vi "Read OPC UA to Azure SQL.vi"() -> ()   [LabVIEW 2019]
uses:
  <vilib>/OPCUA/client/Multiple Read Double.vi
  <vilib>/OPCUA/NI OPC UA Client.lvlib
panel:
  in  "SQL Connection string":string="PROVIDER=SQLOLEDB;DATA SOURCE=tcp:220888.database.windows.net;UID=haavardnk;PWD=Password123;DATABASE=Lab1"
  out "Temperature Value":dbl=24.475354555818342
  in  "Server Endpoint URL":string="opc.tcp://DESKTOP-2K1CGSL:49580"
  in  "stop":bool
  in  "Node Id":string="ns=2;s=Process Data.Temperature"
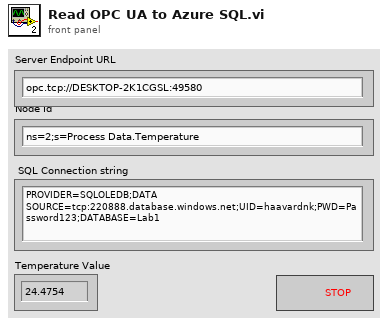
[diagram p1: front panel]
types:
  T1 = cluster{"message mode":enum16{"None", "Sign", "Sign and Encrypt"}, "security":enum16{"Basic256", "Basic128Rsa15"}}
  T2 = typedef "OPC UA Client Refnum.ctl" = refnum<k21>
  T3 = typedef "NodeId.ctl" = string
  T4 = typedef "OPC UA StatusCode.ctl" = u32
  T5 = cluster{"node ID":T3, "value ":dbl, "timestamp":timestamp, "status":T4}[]
  T6 = cluster{"node ID":T3, "value ":dbl, "timestamp":timestamp, "status":T4}
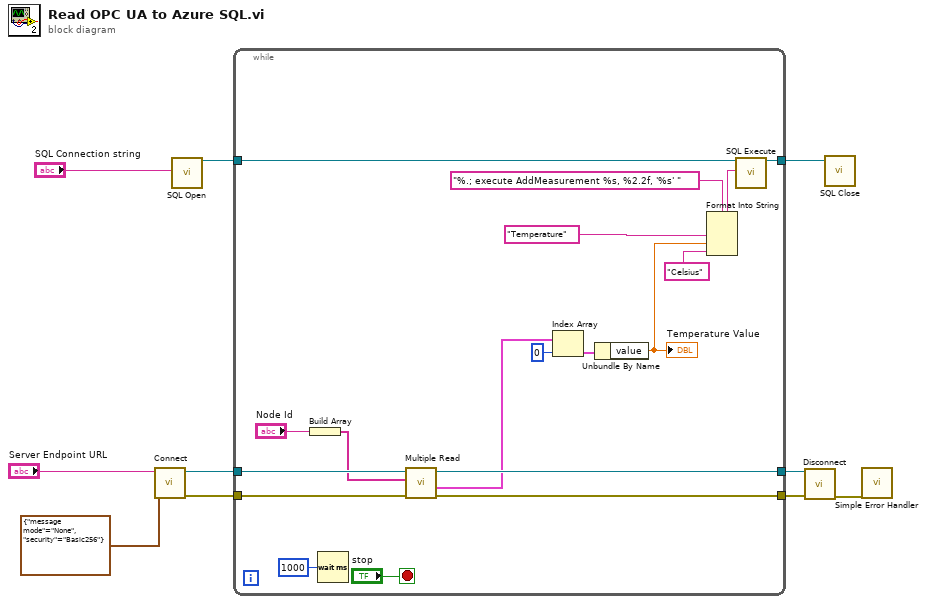
[diagram p0: block diagram]
diagram:
  n1 = call <vilib>:"Connect.vi"("security policy"=T1 {"message mode"=enum."None", "security"=enum."Basic256"}, "server endpoint URL"="Server Endpoint URL") -> ("error out"=w7:errorcluster, "OPC UA client refnum out"=w8:T2)  [unwired: 7 in, 1 out]
  n2 = call <vilib>:"SQL Open.vi"("ConnectionString In"="SQL Connection string") -> ("Connection Out"=w3:refnum<k7>)  [unwired: 17 in, 1 out]
  n3 = while {
    tunnel: w8 -> [w26]
    tunnel: w7 -> [w25]
    tunnel: [w24] -> w5
    tunnel: [w23] -> w6
    tunnel: w3 -> [w16]
    tunnel: [w15] -> w2
    stop <- "stop" stop-if-true
    n4 = Build Array("Node Id") -> (w21:string[])
    n5 = Wait (ms)(milliseconds to wait=u32 1000) -> ()  [unwired: 1 out]
    n6 = call-poly <vilib>:"Multiple Read.vi"("error in (no error)"=w25, "node IDs"=w21, "OPC UA client refnum in"=w26) -> ("error out"=w24:errorcluster, "results"=w20:T5, "OPC UA client refnum out"=w23:T2)  [unwired: 5 in, 1 out]
    n7 = Index Array "Index Array"(array=w20, index=0) -> (element=w18:T6)
    n8 = Unbundle By Name(w18) -> ("value"=w13:dbl)
    "Temperature Value" <- w13
    n9 = Format Into String(format string="%.; execute AddMeasurement %s, %2.2f, '%s' ", "Temperature" ("input 1"), w13, "Celsius" ("input 3")) -> (resulting string=w17:string)  [unwired: 2 in, 1 out]
    n10 = call <vilib>:"SQL Execute.vi"("Connection In"=w16, "SQL Query"=w17) -> ("Connection Out"=w15:refnum<k7>)  [unwired: 16 in, 1 out]
  }
  n11 = call <vilib>:"Disconnect.vi"("error in (no error)"=w5, "OPC UA client refnum in"=w6) -> ("error out"=w4:errorcluster)  [unwired: 9 in]
  n12 = call <vilib>:"SQL Close.vi"("Connection In"=w2) -> ()  [unwired: 18 in, 1 out]
  n13 = call <vilib>:"Simple Error Handler.vi"("error in (no error)"=w4) -> ()  [unwired: 4 in, 5 out]
